vi "Export VI Help.vi"(5 "API Dir":path, 7 "doc dir":path, 8 "error in (no error)":errorcluster, 10 "Language Ring":string(combo)="English(EN)") -> (0 "error out":errorcluster)   [LabVIEW 2017, in "csmdoc.lvlib"]
uses:
  csmdoc.lvlib
  _Shared/CSM Shared.lvlib
  Communicable State Machine.lvlib
  _tool/_file/csm-file-support.lvlib
panel:
  out "Array":path[](array[path])
  out "Numeric":i32=317
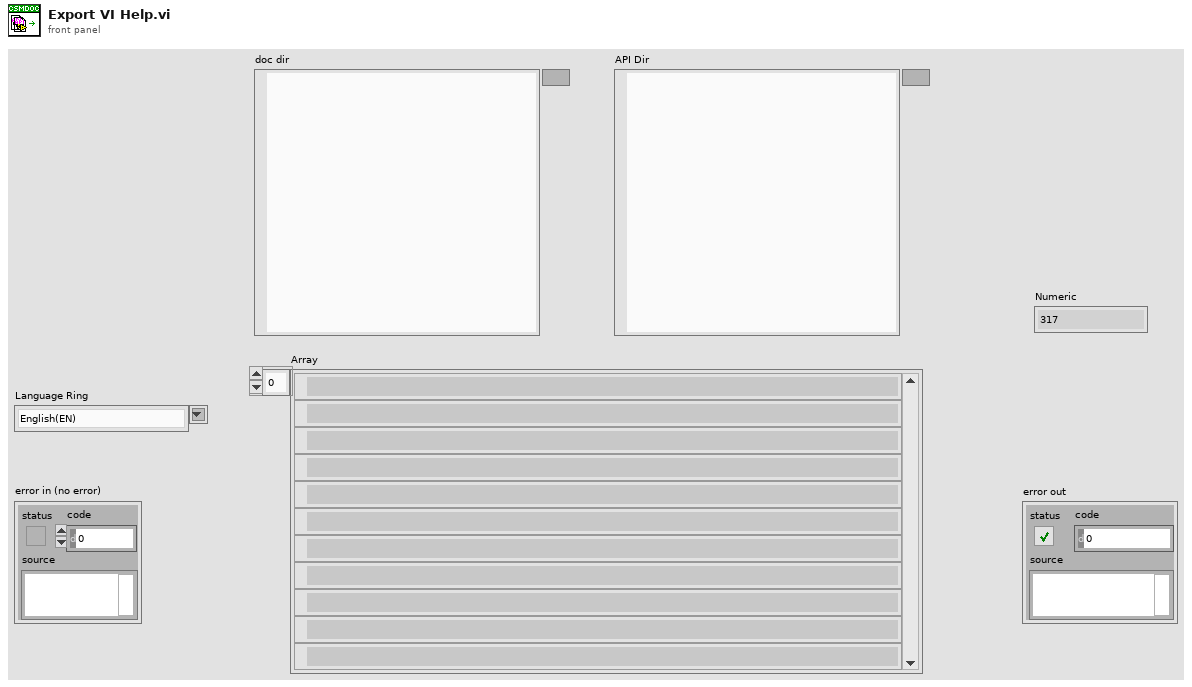
[diagram p1: front panel]
types:
  T1 = typedef "csmdoc.lvlib/DocElement.ctl" = cluster{"ID":string, "Content":string[], "SubIDs":string[], "Path":string[]}
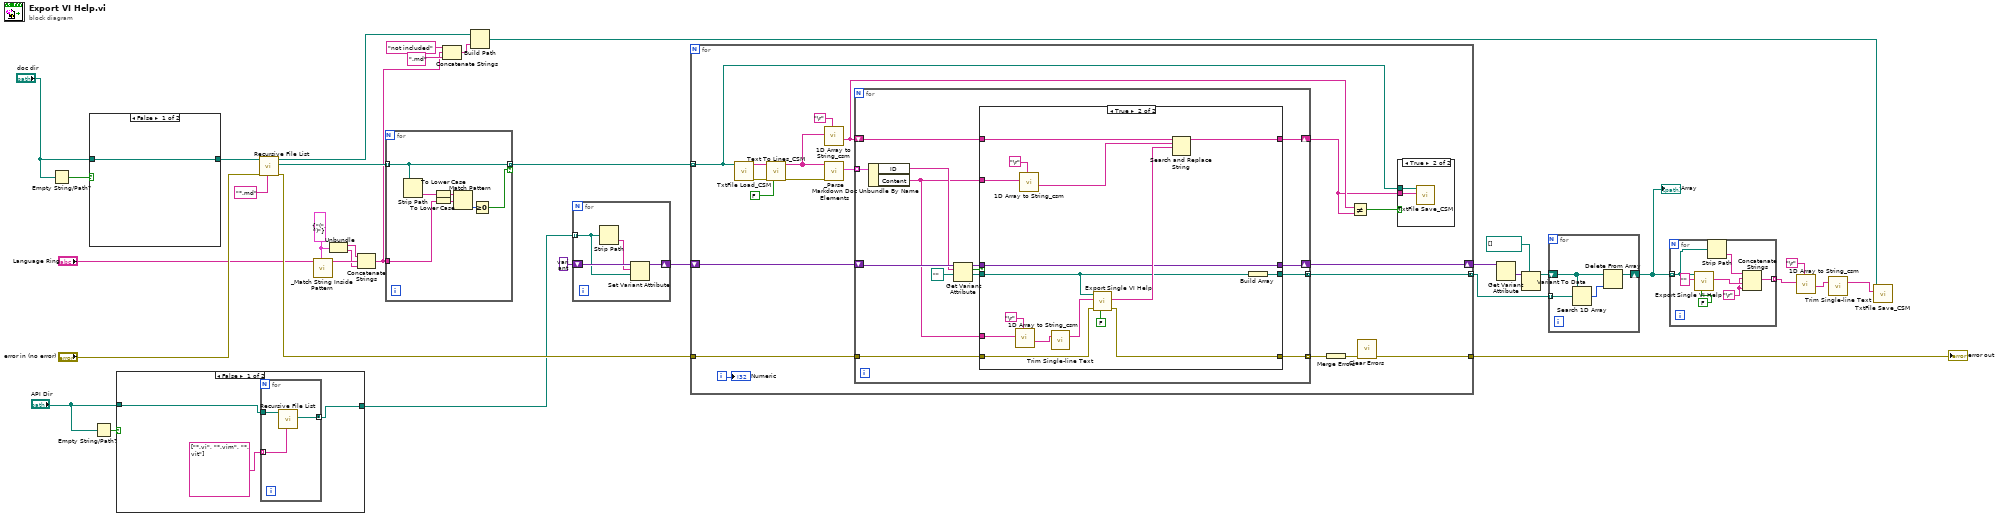
[diagram p0: block diagram]
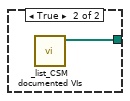
[diagram p2: hidden frame]
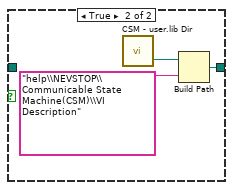
[diagram p3: hidden frame]
diagram:
  w32 = cluster{"left":string, "right":string} {"left"="(", "right"=")"} ("Cluster")
  n1 = Empty String/Path?(string/path="doc dir") -> (empty?=w4:bool)
  n2 = case shown="False" w4 {
    tunnel: [w35 w36] -> w11
    tunnel: "doc dir" -> [w35 _]
    frame False {
    }
    frame True {
      n3 = call "CSM - user.lib Dir.vi"() -> ("<LabVIEW>"=w37:path)  [unwired: 2 in, 1 out]
      n4 = Build Path(base path=w37, name or relative path="help\\NEVSTOP\\Communicable State Machine(CSM)\\VI Description") -> (appended path=w36:path)
    }
  }
  n5 = Empty String/Path?(string/path="API Dir") -> (empty?=w2:bool)
  n6 = case shown="False" w2 {
    tunnel: [w39 w45] -> w25
    tunnel: "API Dir" -> [w40 _]
    frame False {
      n7 = for {
        tunnel: w40 -> [w44]
        tunnel: string[] ["*.vi", "*.vim", "*.vit"] -> [w43] mode=indexing
        tunnel: [w42] -> w39 mode=concatenating
        n8 = call <vilib>:"Recursive File List.vi"("pattern"=w43, "Folder Path"=w44) -> ("All Files in Dir"=w42:path[])  [unwired: 5 in, 4 out]
      }
    }
    frame True {
      n9 = call "_list_CSM documented VIs.vi"() -> ("Array"=w45:path[])  [unwired: 11 in]
    }
  }
  n10 = call <vilib>:"Recursive File List.vi"("pattern"="*.md", "error in (no error)"="error in (no error)", "Folder Path"=w11) -> ("error out"=w26:errorcluster, "All Files in Dir"=w33:path[])  [unwired: 4 in, 3 out]
  n11 = call "_Match String Inside Pattern.vi"("Cluster"=w32, "string"="Language Ring") -> ("String inside"=w31:string)  [unwired: 8 in, 1 out]
  n12 = Unbundle(w32) -> ("left"=w29:string, "right"=w30:string)
  n13 = Concatenate Strings(w29, w31, w30) -> (w7:string)
  n14 = for {
    tunnel: w33 -> [w52] mode=indexing
    tunnel: [w52] -> w22 mode=indexing if=w48
    tunnel: w7 -> [w50]
    n15 = Strip Path(path=w52) -> (name=w51:string)  [unwired: 1 out]
    n16 = To Lower Case(string=w51) -> (all lower case string=w46:string)
    n17 = To Lower Case(string=w50) -> (all lower case string=w47:string)
    n18 = Match Pattern(string=w46, regular expression=w47) -> (offset past match=w49:i32)  [unwired: 1 in, 3 out]
    n19 = Greater Or Equal To 0?(x=w49) -> (x >= 0?=w48:bool)
  }
  n20 = Concatenate Strings("not included" ("string"), w7, ".md" ("string")) -> (w6:string)
  n21 = Build Path(base path=w11, name or relative path=w6) -> (appended path=w5:path)
  n22 = for {
    tunnel: w25 -> [w54] mode=indexing
    shift-right: [w55] -> w23
    shift-left: variant -> [w56]
    n23 = Strip Path(path=w54) -> (name=w53:string)  [unwired: 1 out]
    n24 = Set Variant Attribute(Variant=w56, name=w53, value=w54) -> (Variant out=w55:variant)  [unwired: 1 in, 2 out]
  }
  n25 = for {
    tunnel: w22 -> [w62] mode=indexing
    shift-right: [w64] -> w21
    shift-left: w23 -> [w71]
    tunnel: w26 -> [w75]
    tunnel: [w58] -> w27
    tunnel: [w57] -> w17 mode=concatenating
    i -> [w74]
    n26 = call "TxtFile Load_CSM.vi"("Path"=w62) -> ("error out"=w69:errorcluster, "Text"=w67:string)  [unwired: 9 in]
    n27 = call "Text To Lines_CSM.vi"("Remove Empty Lines? (T)"=FALSE ("Remove Empty Lines?(T)"), "error in (no error)"=w69, "String"=w67) -> ("error out"=w68:errorcluster, "Lines"=w65:string[])  [unwired: 7 in]
    n28 = call "1D Array to String_csm.vi"("delimiter (Tab)"="\r", "Array of Strings"=w65) -> ("delimited string"=w63:string)  [unwired: 9 in]
    n29 = call "_Parse Markdown Doc Elements.vi"("Error in"=w68, "Lines"=w65) -> ("Array"=w72:T1[])  [unwired: 7 in, 2 out]
    n30 = for {
      tunnel: w72 -> [w89] mode=indexing
      shift-right: [w79] -> w64
      shift-left: w71 -> [w88]
      shift-right: [w83] -> w61
      shift-left: w63 -> [w82]
      tunnel: w75 -> [w91]
      tunnel: [w90] -> w73 mode=indexing
      tunnel: [w78] -> w57 mode=concatenating
      n31 = Unbundle By Name(w89) -> ("ID"=w87:string, "Content"=w81:string[])
      n32 = Get Variant Attribute(Variant=w88, name=w87, default value (empty Variant)=path "") -> (duplicate Variant=w80:variant, found=w85:bool, value=w84:path)  [unwired: 1 in, 1 out]
      n33 = case shown="True" w85 {
        tunnel: w91 -> [w94 w110]
        tunnel: [w94 w109] -> w90
        tunnel: w84 -> [_ w96]
        tunnel: w81 -> [_ w104]
        tunnel: [w93 w100] -> w83
        tunnel: w82 -> [w93 w101]
        tunnel: w81 -> [_ w102]
        tunnel: w80 -> [w92 w97]
        tunnel: [w92 w97] -> w79
        tunnel: [_ w95] -> w78
        frame False {
        }
        frame True {
          n34 = call "1D Array to String_csm.vi"("delimiter (Tab)"="\r", "Array of Strings"=w104) -> ("delimited string"=w107:string)  [unwired: 9 in]
          n35 = call "1D Array to String_csm.vi"("delimiter (Tab)"="\r", "Array of Strings"=w102) -> ("delimited string"=w99:string)  [unwired: 9 in]
          n36 = call "Trim Single-line Text.vi"("single-line text"=w107) -> ("trimed text"=w106:string)  [unwired: 2 in]
          n37 = call "Export Single VI Help.vi"("Show FP"=FALSE, "error in (no error)"=w110, "VI Description"=w106, "Path"=w96) -> ("error out"=w109:errorcluster, "VI Description Out"=w98:string)  [unwired: 6 in]
          n38 = Search and Replace String(input string=w101, search string=w99, replace string=w98) -> (result string=w100:string)  [unwired: 5 in, 3 out]
          n39 = Build Array(w96) -> (w95:path[])
        }
      }
    }
    n40 = Merge Errors(w73) -> (w59:errorcluster)
    n41 = Not Equal?(x=w63, y=w61) -> (x != y?=w60:bool)
    n42 = call <vilib>:"Clear Errors.vi"("error in (no error)"=w59) -> ("error out"=w58:errorcluster)  [unwired: 5 in, 1 out]
    n43 = case shown="True" w60 {
      tunnel: w62 -> [_ w77]
      tunnel: w61 -> [_ w76]
      frame False {
      }
      frame True {
        n44 = call "TxtFile Save_CSM.vi"("text"=w76, "Path"=w77) -> ()  [unwired: 9 in, 1 out]
      }
    }
    "Numeric" <- w74
  }
  "error out" <- w27
  n45 = Get Variant Attribute(Variant=w21) -> (values=w20:variant[])  [unwired: 3 in, 3 out]
  n46 = Variant To Data(type=path[] [], Variant=w20) -> (data=w18:path[])  [unwired: 1 in, 1 out]
  n47 = for {
    shift-right: [w111] -> w16
    shift-left: w18 -> [w112]
    tunnel: w17 -> [w114] mode=indexing
    n48 = Search 1D Array(1D array=w112, element=w114) -> (index of element=w113:i32)  [unwired: 1 in]
    n49 = Delete From Array(array=w112, index=w113) -> (array with subset deleted=w111:path[])  [unwired: 1 in, 1 out]
  }
  "Array" <- w16
  n50 = for {
    tunnel: w16 -> [w116] mode=indexing
    tunnel: [w118] -> w13 mode=indexing
    w117 = "\r"
    n51 = call "Export Single VI Help.vi"("Show FP"=FALSE, "VI Description"="", "Path"=w116) -> ("VI Description Out"=w120:string)  [unwired: 7 in, 1 out]
    n52 = Strip Path(path=w116) -> (name=w115:string)  [unwired: 1 out]
    n53 = Concatenate Strings(w115, w117, w120, w117) -> (w118:string)
  }
  n54 = call "1D Array to String_csm.vi"("delimiter (Tab)"="\r", "Array of Strings"=w13) -> ("delimited string"=w15:string)  [unwired: 9 in]
  n55 = call "Trim Single-line Text.vi"("single-line text"=w15) -> ("trimed text"=w12:string)  [unwired: 2 in]
  n56 = call "TxtFile Save_CSM.vi"("text"=w12, "Path"=w5) -> ()  [unwired: 9 in, 1 out]
